vi "GetVersion.vi"(4 "error in (no error)":errorcluster, 7 "axis in":cluster{"keyHandle":u32, "nodeId":u16}={"keyHandle"=0, "nodeId"=1}) -> (0 "error out":errorcluster, 2 "version numbers":T1 {"applicationVersion" format="%x"; "applicationNumber" format="%x"; "softwareVersion" format="%x"; "hardwareVersion" format="%x"}, 3 "axis out":cluster{"keyHandle":u32, "nodeId":u16}={"keyHandle"=0, "nodeId"=1})   [LabVIEW 2017, in "maxonEPOS.lvlib"]
doc: "<B>GetVersion</B> returns the firmware version (software version, hardware version, application number, application version)."
uses:
  Examples/maxonEPOS.lvlib
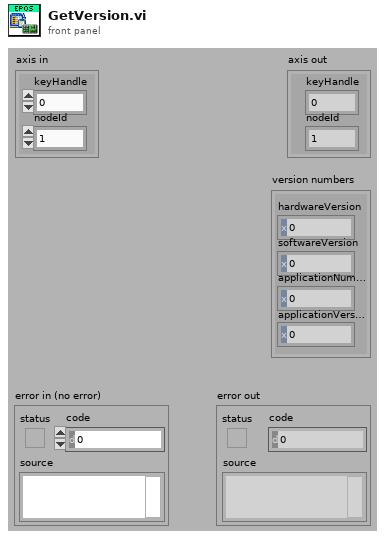
[diagram p1: front panel]
types:
  T1 = cluster{"hardwareVersion ":u16, "softwareVersion ":u16, "applicationNumber":u16, "applicationVersion":u16}
  T2 = cluster{"hardwareVersion":u16, "softwareVersion":u16, "applicationNumber":u16, "applicationVersion":u16}
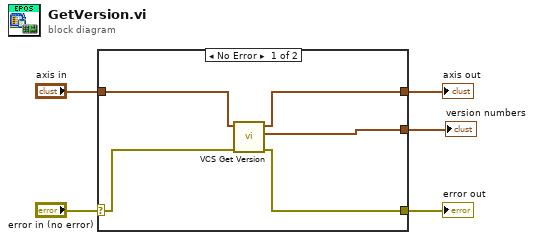
[diagram p0: block diagram]
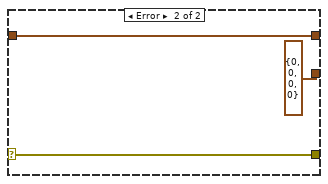
[diagram p2: hidden frame]
diagram:
  n1 = case shown="No Error" "error in (no error)" {
    selector: "error in (no error)" -> [w6 w13]
    tunnel: [w9 w13] -> w4
    tunnel: [w10 w12] -> w3
    tunnel: "axis in" -> [w7 w12]
    tunnel: [w8 T2 {"hardwareVersion"=0, "softwareVersion"=0, "applicationNumber"=0, "applicationVersion"=0} ("version numbers")] -> w1
    frame No Error {
      n2 = call "VCS Get Version.vi"("error in (no error)"=w6, "axis In"=w7) -> ("error out"=w9:errorcluster, "version numbers"=w8:T1, "axis Out"=w10:cluster{"keyHandle":u32, "nodeId":u16})  [unwired: 7 in]
    }
    frame Error {
    }
  }
  "error out" <- w4
  "axis out" <- w3
  "version numbers" <- w1
